vi "Arrange Array.vi"(1 "Order":string[](array[string]), 2 "Array to Arrange":T1(array[cluster])) -> (0 "Arranged Array":T1(array[cluster]))   [LabVIEW 2011]
doc: "This VI arranges an array in a specific order based on each element's name."
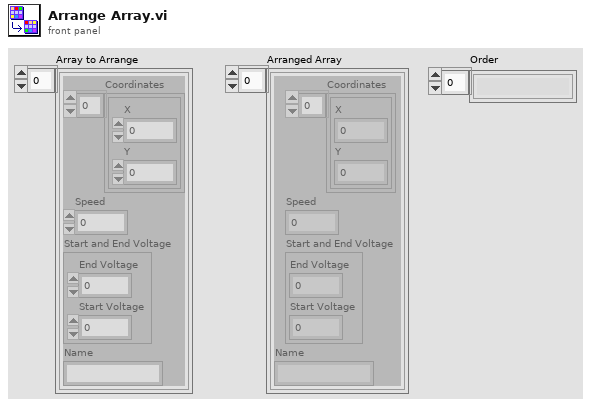
[diagram p1: front panel]
types:
  T1 = cluster{"Coordinates":cluster{"X":dbl, "Y":dbl}[], "Speed":dbl, "Start and End Voltage":cluster{"End Voltage":dbl, "Start Voltage":dbl}, "Name":string}[]
  T2 = cluster{"Coordinates":cluster{"X":dbl, "Y":dbl}[], "Speed":dbl, "Start and End Voltage":cluster{"End Voltage":dbl, "Start Voltage":dbl}, "Name":string}
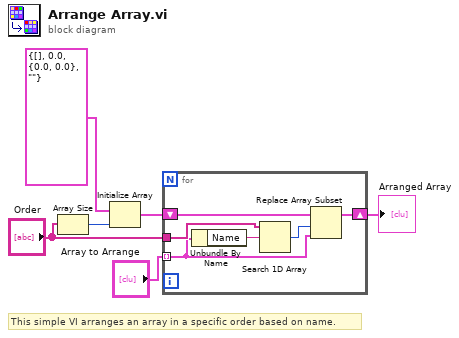
[diagram p0: block diagram]
diagram:
  # "This simple VI arranges an array in a specific order based on name."
  n1 = Array Size(array="Order") -> (size(s)=w5:i32)
  n2 = Initialize Array(T2 {"Coordinates"=[], "Speed"=0.0, "Start and End Voltage"={"End Voltage"=0.0, "Start Voltage"=0.0}, "Name"=""}, w5) -> (w3:T1)
  n3 = for {
    tunnel: "Array to Arrange" -> [w9] mode=indexing
    tunnel: "Order" -> [w11]
    shift-right: [w8] -> w1
    shift-left: w3 -> [w7]
    n4 = Unbundle By Name(w9) -> ("Name"=w10:string)
    n5 = Search 1D Array(1D array=w11, element=w10) -> (index of element=w12:i32)  [unwired: 1 in]
    n6 = Replace Array Subset(array=w7, new element=w9, index=w12) -> (w8:T1)
  }
  "Arranged Array" <- w1
